vi "Charact One Point.vi"(0 "SG SC2250 Path in":refnum<class "SG SC2250 Path.lvclass">, 5 "Cal point in":T1, 11 "error in (no error)":errorcluster) -> (4 "SG SC2250 Path out":refnum<class "SG SC2250 Path.lvclass">, 15 "error out":errorcluster)   [LabVIEW 2023, in "RFFixtureCharact.RFPM.lvlib" / "SG SC2250 Path.lvclass"]
uses:
  SG SC2250 Path.lvclass
  C:/srd-semi-rfcal-software/AuxTools/STSRFFixtureCharactUtility/Source/Code Modules/Common/Base Classes/Path/Path.lvclass
  Public/Base Classes/Scalar/Scalar Path/Type Definitions/Cal Point.ctl
  Public/Base Classes/Scalar/Scalar Path/Type Definitions/Scalar Charact Result.ctl
  SG SC2250 Path.lvclass/SG SC2250 Path.ctl
  Properties/Read SC2250 Session.vi
  Public/Base Classes/Scalar/Scalar Path/Scalar Path.lvclass
  Public/RFFixtureCharact.Public.lvlib
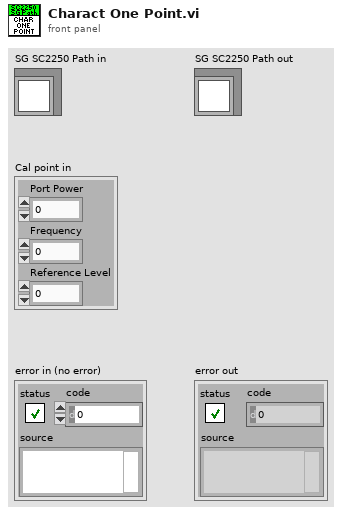
[diagram p1: front panel]
types:
  T1 = typedef "RFFixtureCharact.Public.lvlib/Scalar Path.lvclass/Cal Point.ctl" = cluster{"Port Power":dbl, "Frequency":dbl, "Reference Level":dbl}
  T2 = typedef "RFFixtureCharact.Public.lvlib/Scalar Path.lvclass/Scalar Charact Result.ctl" = cluster{"Port Power":dbl, "Reference Level":dbl, "Frequency":dbl, "Path Gain":dbl, "Out Of Limit":bool}
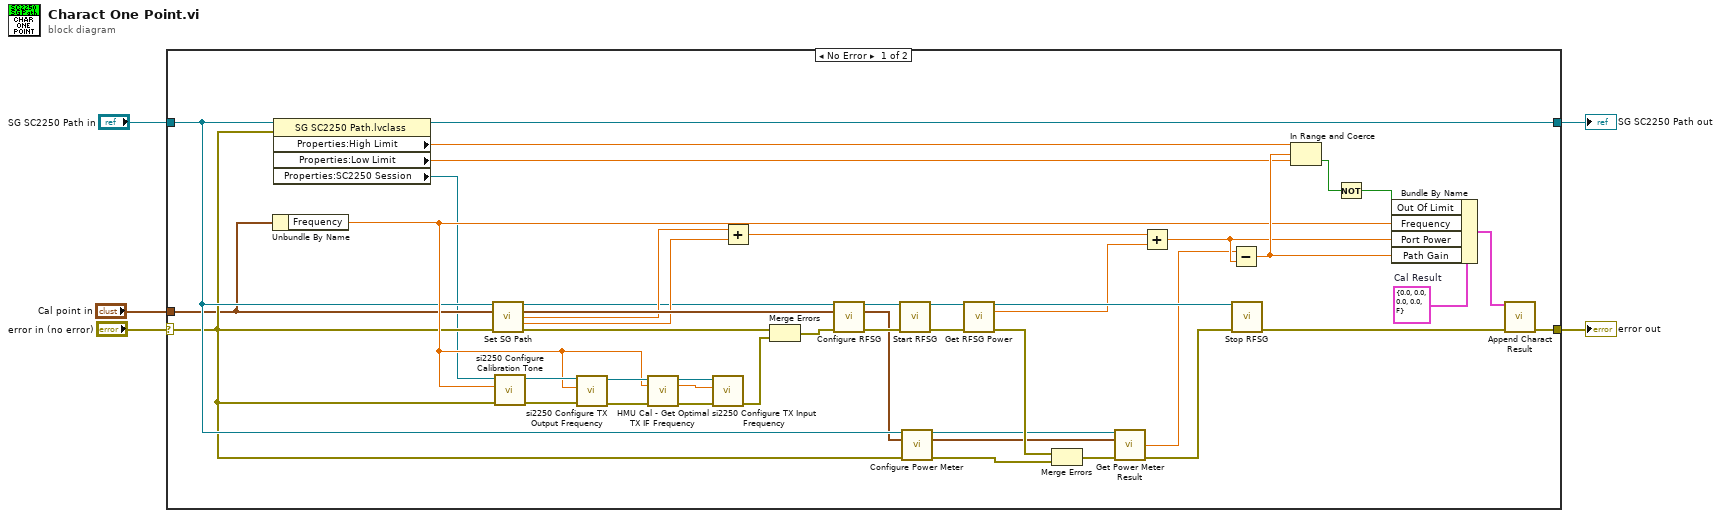
[diagram p0: block diagram]
diagram:
  n1 = case shown="No Error" "error in (no error)" {
    selector: "error in (no error)" -> [w18 w51]
    tunnel: "SG SC2250 Path in" -> [w20 w50]
    tunnel: "Cal point in" -> [w16 _]
    tunnel: [w36 w51] -> w5
    tunnel: [w39 w50] -> w1
    frame No Error {
      w45 = T2 {"Port Power"=0.0, "Reference Level"=0.0, "Frequency"=0.0, "Path Gain"=0.0, "Out Of Limit"=FALSE}  # Cal Result
      n2 = Unbundle By Name(w16) -> ("Frequency"=w23:dbl)
      n3 = property class="SG SC2250 Path.lvclass"(reference=w20, error in=w18) -> (reference out=w39:refnum<class "SG SC2250 Path.lvclass">, "Properties:High Limit"=w41:dbl, "Properties:Low Limit"=w40:dbl, "Properties:SC2250 Session"=w10:refnum<k15>)  [unwired: 1 out]
      n4 = call-dynamic "Set SG Path.vi"("Scalar SG Si2250 Path in"=w20, "Cal point in"=w16, "error in (no error)"=w18) -> ("Scalar SG Si2250 Path out"=w9:refnum<class "SG SC2250 Path.lvclass">, "Cal point out"=w48:T1, "Source Gain"=w13:dbl, "Digital Gain"=w11:dbl, "error out"=w26:errorcluster)  [unwired: 8 in]
      n5 = call <instrlib>:"si2250 Configure Calibration Tone.vi"("error in"=w18, "Output Frequency"=w23, "instrument handle"=w10) -> ("error out"=w34:errorcluster, "instrument handle out"=w33:refnum<k15>)  [unwired: 6 in, 1 out]
      n6 = call <instrlib>:"si2250 Configure TX Output Frequency.vi"("error in"=w34, "Output Frequency"=w23, "instrument handle"=w33) -> ("error out"=w30:errorcluster, "instrument handle out"=w31:refnum<k15>)  [unwired: 7 in]
      n7 = call "HMU Cal - Get Optimal TX IF Frequency.vi"("RF Frequency (Hz)"=w23, "error in (no error)"=w30) -> ("IF Frequency (Hz)"=w29:dbl, "error out"=w32:errorcluster)  [unwired: 12 in]
      n8 = call <instrlib>:"si2250 Configure TX Input Frequency.vi"("error in"=w32, "Input Frequency"=w29, "instrument handle"=w31) -> ("error out"=w27:errorcluster)  [unwired: 7 in, 1 out]
      n9 = Add(x=w13, y=w11) -> (x+y=w12:dbl)
      n10 = Merge Errors(w26, w27) -> (w25:errorcluster)
      n11 = call-dynamic "Configure RFSG.vi"("Scalar SG Si2250 Path in"=w9, "Cal point in"=w48, "error in (no error)"=w25) -> ("Scalar SG Si2250 Path out"=w8:refnum<class "SG SC2250 Path.lvclass">, "Cal point out"=w15:T1, "error out"=w49:errorcluster)  [unwired: 10 in]
      n12 = call-dynamic "Start RFSG.vi"("Path in"=w8, "error in (no error)"=w49) -> ("Path out"=w46:refnum<class "SG SC2250 Path.lvclass">, "error out"=w47:errorcluster)  [unwired: 12 in]
      n13 = call-dynamic "Configure Power Meter.vi"("SG Path in"=w20, "Cal point in"=w15, "error in (no error)"=w18) -> ("SG Path out"=w19:refnum<class "SG SC2250 Path.lvclass">, "Cal point out"=w14:T1, "error out"=w17:errorcluster)  [unwired: 10 in]
      n14 = call-dynamic "Get RFSG Power.vi"("Path in"=w46, "error in (no error)"=w47) -> ("Path out"=w38:refnum<class "SG SC2250 Path.lvclass">, "Power Level (dBm)"=w28:dbl, "error out"=w24:errorcluster)  [unwired: 11 in]
      n15 = Merge Errors(w24, w17) -> (w22:errorcluster)
      n16 = call-dynamic "Get Power Meter Result.vi"("SG Path in"=w19, "Cal point in"=w14, "error in (no error)"=w22) -> ("Power (dBm)"=w6:dbl, "error out"=w21:errorcluster)  [unwired: 10 in, 1 out]
      n17 = Add(x=w12, y=w28) -> (x+y=w7:dbl)
      n18 = Subtract(x=w6, y=w7) -> (x-y=w42:dbl)
      n19 = call-dynamic "Stop RFSG.vi"("Path in"=w38, "error in (no error)"=w21) -> ("error out"=w37:errorcluster)  [unwired: 12 in, 1 out]
      n20 = In Range and Coerce(upper limit=w41, x=w42, lower limit=w40) -> (In Range?=w43:bool)  [unwired: 1 out]
      n21 = Not(x=w43) -> (.not. x?=w44:bool)
      n22 = Bundle By Name(cluster=w45, "Out Of Limit"=w44, "Frequency"=w23, "Port Power"=w7, "Path Gain"=w42) -> (w35:T2)
      n23 = call "Append Charact Result.vi"("Path cal resut in"=w35, "error in (no error)"=w37) -> ("error out"=w36:errorcluster)  [unwired: 13 in]
    }
    frame Error {
    }
  }
  "error out" <- w5
  "SG SC2250 Path out" <- w1
